vi "Compensation.VI"(0 "VISA resource name":refnum<visa-resource-name>, 1 "Single Freq (F:All Freq)":bool, 2 "Frequency Point (1)":enum16{"1", "2", "3"}(ring)=enum."2", 3 "Compensation (0:OPEN)":enum16{"OPEN", "SHORT", "LOAD"}(ring), 5 "OPEN (F:OFF)":bool, 7 "SHORT (F:OFF)":bool, 9 "LOAD (F:OFF)":bool, 11 "error in (no error)":errorcluster) -> (4 "VISA resource name out":refnum<visa-resource-name>, 15 "error out":errorcluster)   [LabVIEW 2016, in "Agilent 428X Series.lvlib"]
doc: "This VI is to handle the OPEN, SHORT, and LOAD compensation for the instrument. User can select for single frequency/ all frequency mode. \n\nWARNING: This VI contains a pop up dialog box it will require modification if you wish to be able to use this VI without user intervention."
uses:
  <instrlib>/Agilent 428X Series/Agilent 428X Series.lvlib
panel:
  # "WARNING: Model 4284 Only!  \nThis VI contains a pop up dialog box it will require modification \nif you wish to be able to use this VI without user intervention."
  # "ON\nOFF"
  # "ON\nOFF"
  # "ON\nOFF"
  # ":"
  # "SINGLE\nALL"
  # "Needs to include beep and instruction to operator\nto connect Open, Short, or Load."
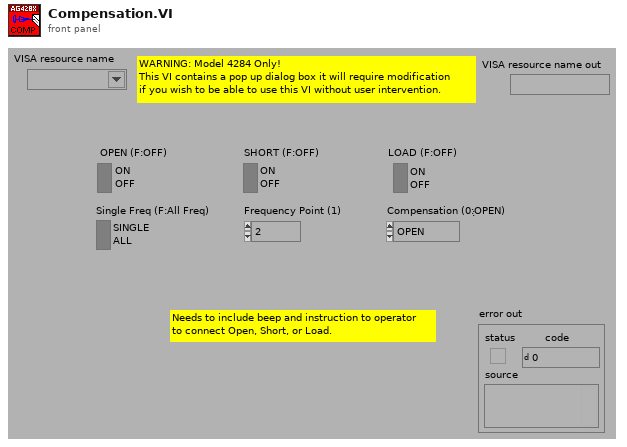
[diagram p1: front panel]
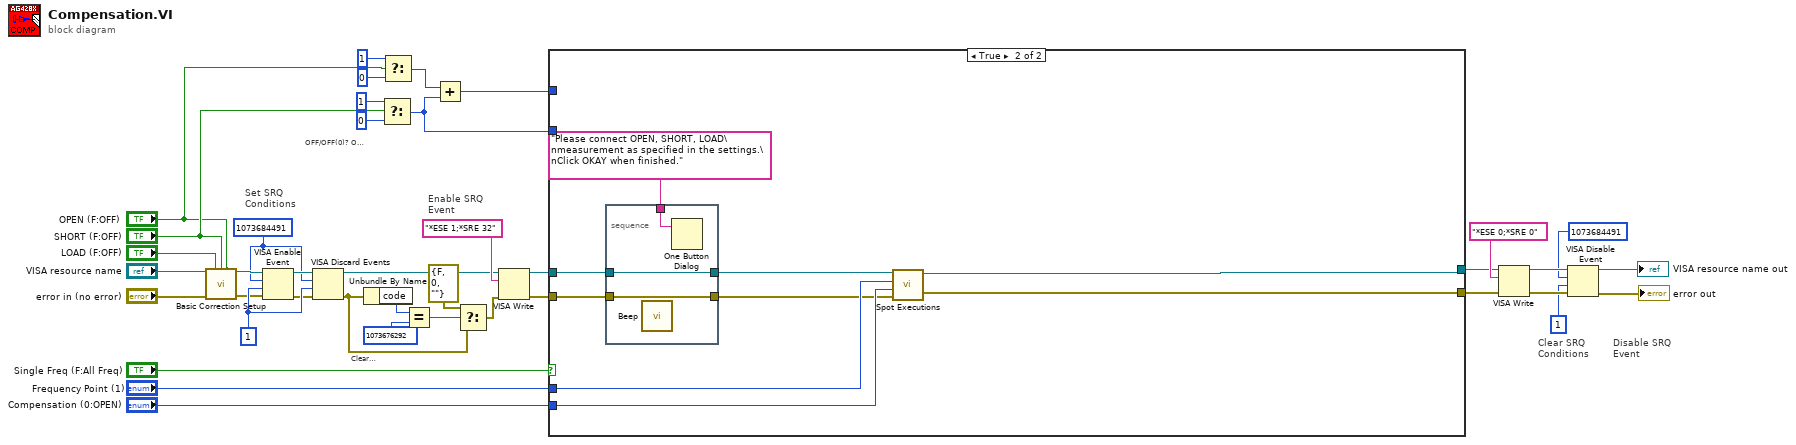
[diagram p0: block diagram]
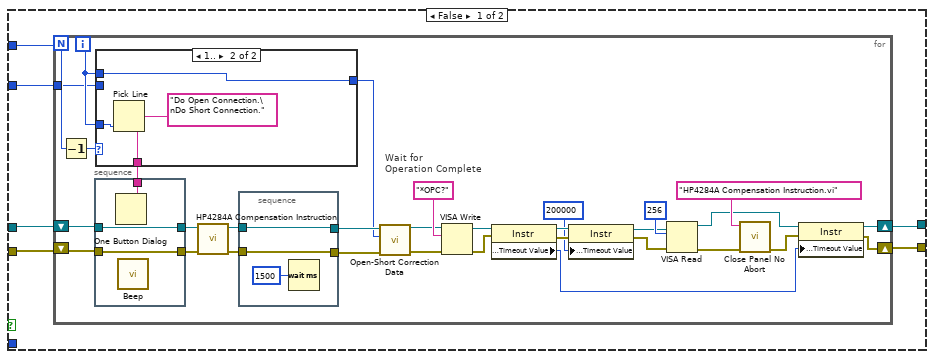
[diagram p2: hidden frame]
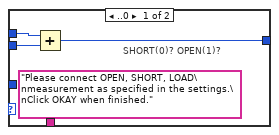
[diagram p3: hidden frame]
diagram:
  w37 = u16 1
  w25 = u32 1073684491
  # "OFF/OFF(0)? ON/OFF(1)? ON/ON(2)?"
  # "Clear Warning Codes"
  # "Disable SRQ \nEvent"
  # "Clear SRQ\nConditions"
  # "Set SRQ\nConditions"
  # "Enable SRQ \nEvent"
  n1 = call <instrlib>:"Basic Correction Setup.vi"("VISA resource name"="VISA resource name", "Load Corr  (F: Off)"="LOAD (F:OFF)", "Short Corr (T: On)"="SHORT (F:OFF)", "Open Corr  (F: Off)"="OPEN (F:OFF)", "error in (no error)"="error in (no error)") -> ("VISA resource name out"=w36:refnum<visa-resource-name>, "error out"=w35:errorcluster)  [unwired: 8 in, 1 out]
  n2 = VISA Enable Event(8:w35, 9:w37, 10:w25, 11:w36) -> (0:w27:errorcluster, 3:w28:refnum<visa-resource-name>)
  n3 = VISA Discard Events(8:w27, 9:w37, 10:w25, 11:w28) -> (0:w15:errorcluster, 3:w26:refnum<visa-resource-name>)
  n4 = Unbundle By Name(w15) -> ("code"=w18:i32)
  n5 = Select(t=i8 1, s="SHORT (F:OFF)", f=i8 0) -> (s? t:f=w4:i8)
  n6 = Select(t=i8 1, s="OPEN (F:OFF)", f=i8 0) -> (s? t:f=w5:i8)
  n7 = Equal?(x=w18, y=1073676292) -> (x = y?=w16:bool)
  n8 = Add(x=w5, y=w4) -> (x+y=w7:i8)
  n9 = Select(t=errorcluster {"status"=FALSE, "code"=0, "source"=""} ("error out"), s=w16, f=w15) -> (s? t:f=w12:errorcluster)
  n10 = VISA Write(VISA resource name=w26, write buffer="*ESE 1;*SRE 32" ("write buffer (\"\")"), error in (no error)=w12) -> (VISA resource name out=w34:refnum<visa-resource-name>, error out=w13:errorcluster)  [unwired: 1 out]
  n11 = case shown="True" "Single Freq (F:All Freq)" {
    tunnel: w34 -> [w41 w96]
    tunnel: w13 -> [w44 w94]
    tunnel: [w42 w101] -> w1
    tunnel: [w43 w100] -> w6
    tunnel: "Frequency Point (1)" -> [_ w99]
    tunnel: "Compensation (0:OPEN)" -> [_ w98]
    tunnel: w7 -> [w46 _]
    tunnel: w4 -> [w45 _]
    frame False {
      n12 = for {
        N: w46 -> [w57]
        tunnel: w45 -> [w54]
        shift-right: [w51] -> w43
        shift-left: w44 -> [w53]
        shift-right: [w50] -> w42
        shift-left: w41 -> [w49]
        i -> [w58]
        # "Wait for \nOperation Complete"
        n13 = Decrement(x=w57) -> (x-1=w56:i32)
        n14 = case shown="1.." w56 {
          tunnel: ["Please connect OPEN, SHORT, LOAD\nmeasurement as specified in the settings.\nClick OKAY when finished." w85] -> w76
          tunnel: w58 -> [_ w84]
          tunnel: w58 -> [w81 w83]
          tunnel: [w80 w83] -> w55
          tunnel: w54 -> [w79 _]
          frame ..0 {
            # "SHORT(0)? OPEN(1)?"
            n15 = Add(x=w81, y=w79) -> (x+y=w80:i32)
          }
          frame 1.. {
            n16 = Pick Line(multi-line string="Do Open Connection.\nDo Short Connection.", line index=w84) -> (output string=w85:string)  [unwired: 1 in]
          }
        }
        n17 = stacked-sequence {
          tunnel: w49 -> [w89]
          tunnel: [w89] -> w62
          tunnel: w53 -> [w88]
          tunnel: [w88] -> w60
          tunnel: w76 -> [w87]
          frame #0 {
            n18 = One Button Dialog(message=w87) -> ()  [unwired: 1 in, 1 out]
            n19 = call <vilib>:"Beep.vi"() -> ()  [unwired: 12 in]
          }
        }
        n20 = call <instrlib>:"HP4284A Compensation Instruction.vi"("error in (no error)"=w60, "VISA resource name"=w62) -> ("error out"=w59:errorcluster, "VISA resource name out"=w61:refnum<visa-resource-name>)  [unwired: 8 in]
        n21 = stacked-sequence {
          tunnel: [w91] -> w64
          tunnel: [w90] -> w63
          tunnel: w61 -> [w91]
          tunnel: w59 -> [w90]
          frame #0 {
            n22 = Wait (ms)(milliseconds to wait=u32 1500) -> ()  [unwired: 1 out]
          }
        }
        n23 = call <instrlib>:"Open-Short Correction Data.vi"("error in (no error)"=w63, "Correction Mode (1: Open)"=w55, "VISA resource name"=w64) -> ("error out"=w67:errorcluster, "VISA resource name out"=w68:refnum<visa-resource-name>)  [unwired: 7 in]
        n24 = VISA Write(VISA resource name=w68, write buffer="*OPC?" ("write buffer (\"\")"), error in (no error)=w67) -> (VISA resource name out=w65:refnum<visa-resource-name>, error out=w66:errorcluster)  [unwired: 1 out]
        n25 = property class="Instr"(reference=w65, error in=w66) -> (reference out=w71:refnum<visa-resource-name>, error out=w72:errorcluster, "General Settings:Timeout Value"=w52:u32)
        n26 = property class="Instr"(reference=w71, error in=w72, "General Settings:Timeout Value"=u32 200000) -> (reference out=w73:refnum<visa-resource-name>, error out=w74:errorcluster)
        n27 = VISA Read(VISA resource name=w73, byte count=u32 256 ("byte count (0)"), error in (no error)=w74) -> (VISA resource name out=w47:refnum<visa-resource-name>, error out=w78:errorcluster)  [unwired: 2 out]
        n28 = call <vilib>:"Close Panel No Abort.vi"("error in (no error)"=w78, "VI name"="HP4284A Compensation Instruction.vi") -> ("error out"=w48:errorcluster)  [unwired: 9 in]
        n29 = property class="Instr"(reference=w47, error in=w48, "General Settings:Timeout Value"=w52) -> (reference out=w50:refnum<visa-resource-name>, error out=w51:errorcluster)
      }
    }
    frame True {
      n30 = stacked-sequence {
        tunnel: "Please connect OPEN, SHORT, LOAD\nmeasurement as specified in the settings.\nClick OKAY when finished." -> [w104]
        tunnel: w96 -> [w103]
        tunnel: [w103] -> w95
        tunnel: w94 -> [w102]
        tunnel: [w102] -> w93
        frame #0 {
          n31 = call <vilib>:"Beep.vi"() -> ()  [unwired: 12 in]
          n32 = One Button Dialog(message=w104) -> ()  [unwired: 1 in, 1 out]
        }
      }
      n33 = call <instrlib>:"Spot Executions.vi"("error in (no error)"=w93, "Mode (0: Open)"=w98, "Spot Number (1)"=w99, "VISA resource name"=w95) -> ("error out"=w100:errorcluster, "VISA resource name out"=w101:refnum<visa-resource-name>)  [unwired: 6 in]
    }
  }
  n34 = VISA Write(VISA resource name=w1, write buffer="*ESE 0;*SRE 0" ("write buffer (\"\")"), error in (no error)=w6) -> (VISA resource name out=w24:refnum<visa-resource-name>, error out=w23:errorcluster)  [unwired: 1 out]
  n35 = VISA Disable Event(8:w23, 9:u16 1, 10:u32 1073684491, 11:w24) -> (0:→"error out":errorcluster, 3:→"VISA resource name out":refnum<visa-resource-name>)
